vi "AB_Get Current VI Settings.vi"(11 "linkerInfo":T4) -> (3 "sourceProperties":T1[](array[typedef]))   [LabVIEW 2020]
uses:
  <vilib>/Utility/lvfile.llb/LVFileType.ctl
  <vilib>/AppBuilder/AB_Source_Properties.ctl
  <vilib>/AppBuilder/AB_Source_Property_Type.ctl
  <vilib>/AppBuilder/AB_Source_Property_WindowBehavior.ctl
  <vilib>/AppBuilder/AB_Source_Property_WindowRunTimePosition.ctl
  <vilib>/Utility/lvfile.llb/NI_FileType.lvlib
panel:
  in  "use hints for keep panel? (T)":bool=TRUE
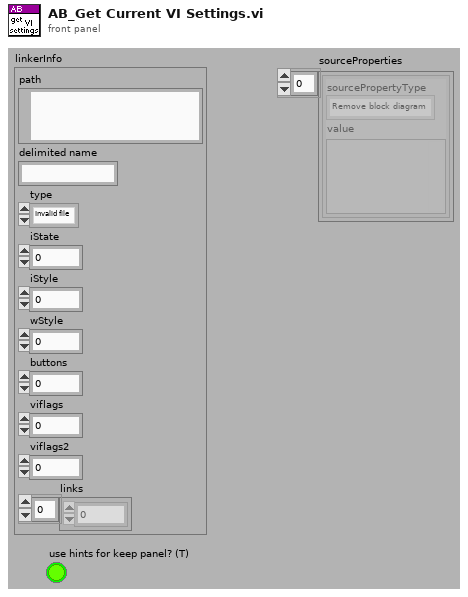
[diagram p1: front panel]
types:
  T1 = typedef "AB_Source_Properties.ctl" = cluster{"sourcePropertyType":T2, "value":variant}
  T2 = typedef "AB_Source_Property_Type.ctl" = enum16{"Remove block diagram", "Remove front panel", "Password", "Window has title bar", "Show menu bar", "Show vertical scroll bar", "Show horizontal scroll bar", "Show toolbar", "Show Abort button", "Show fp when called", "Window behavior", "Allow user to close window", "Window run-time position", "Run when opened", "Allow debugging", "Auto error handling", "Generate guard code", "Use stack variables", "Expression folding", "Integer only", "Inline subVI"}
  T3 = typedef "NI_FileType.lvlib/LVFileType.ctl" = enum32{"Invalid file", "Unknown type", "Instrument", "Control", "Polymorphic VI", "Project", "Library", "LVClass", "XControl", "XNode", "Shared library", ".NET assembly", "ActiveX interface", "CIN", "Run-time menu", "Palette menu", "Help file", "LLB", "XNode Edit Dependency", "Class Private Data Control", "Statechart", "MathScript .m file", "Ladder Diagram", "LVLibp", "XNode Build Dependency"}
  T4 = cluster{"path":path, "delimited name":string, "type":T3, "iState":u32, "iStyle":u16, "wStyle":u16, "buttons":u16, "viflags":u32, "viflags2":u32, "links":u32[]}
  T5 = typedef "AB_Source_Property_WindowBehavior.ctl" = enum16{"Default", "Floating", "Modal"}
  T6 = typedef "AB_Source_Property_WindowRunTimePosition.ctl" = enum16{"Unchanged", "Centered", "Maximized", "Minimized"}
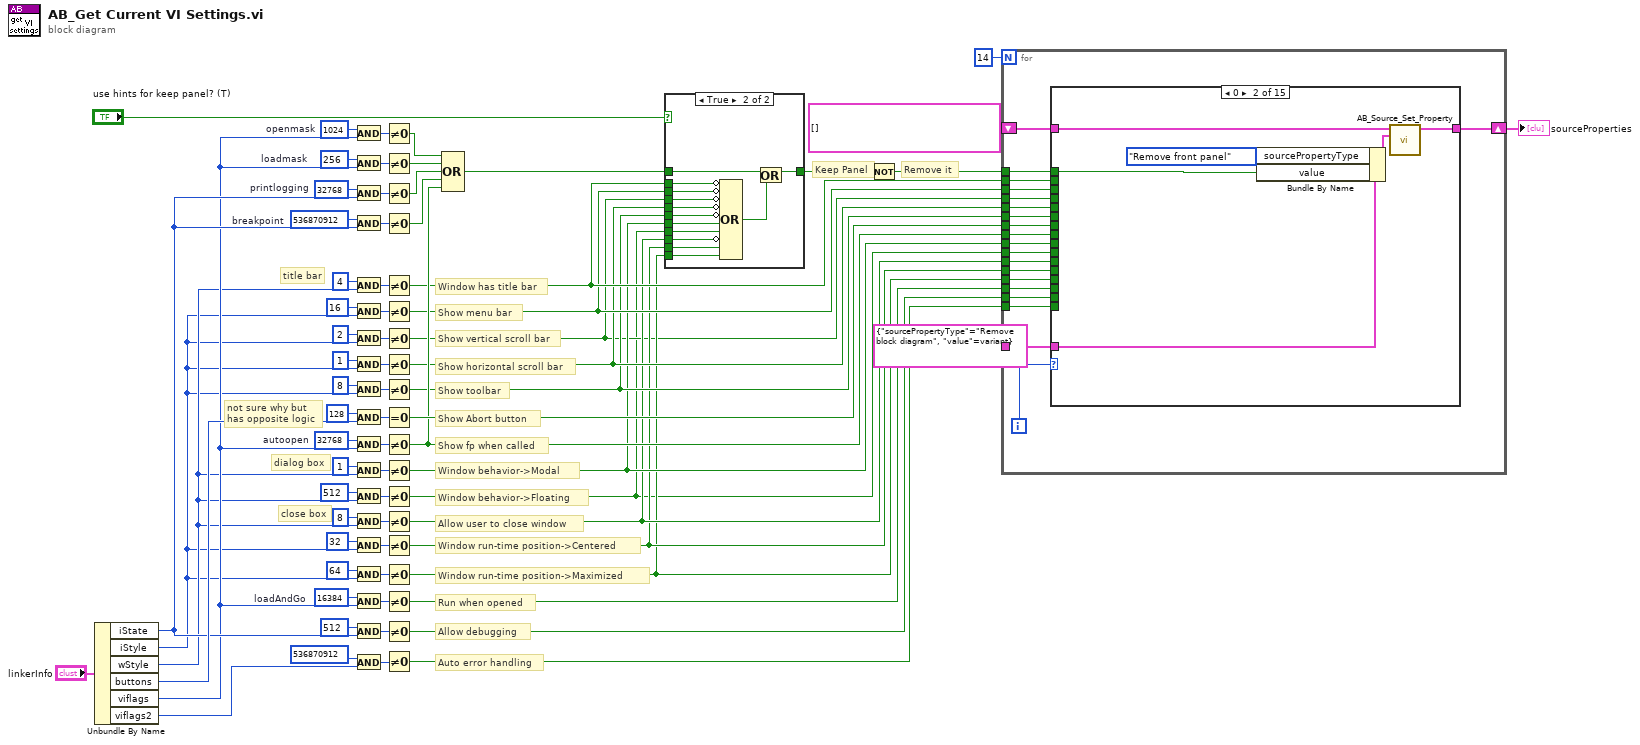
[diagram p0: block diagram]
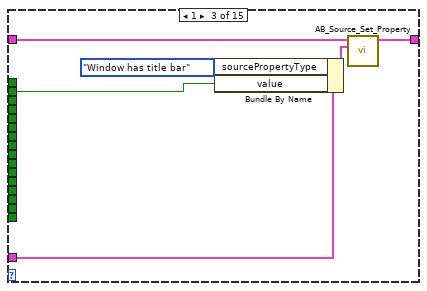
[diagram p3: hidden frame]
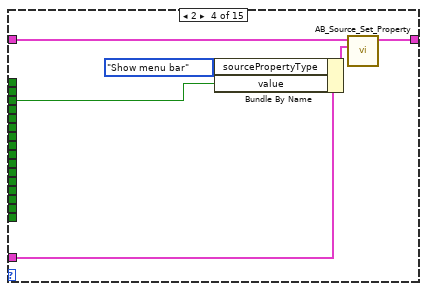
[diagram p4: hidden frame]
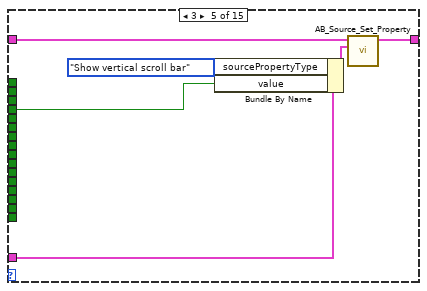
[diagram p5: hidden frame]
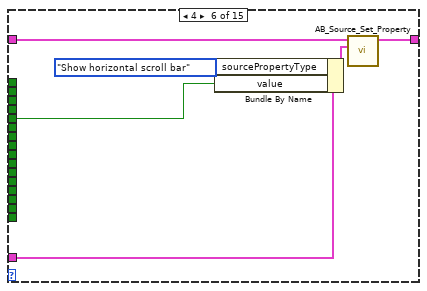
[diagram p6: hidden frame]
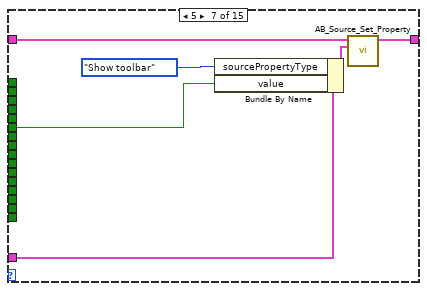
[diagram p7: hidden frame]
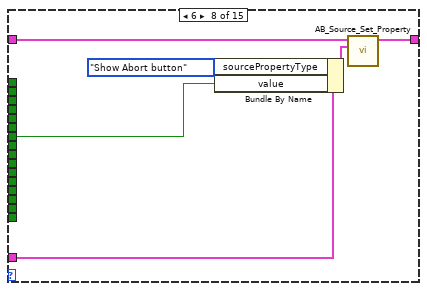
[diagram p8: hidden frame]
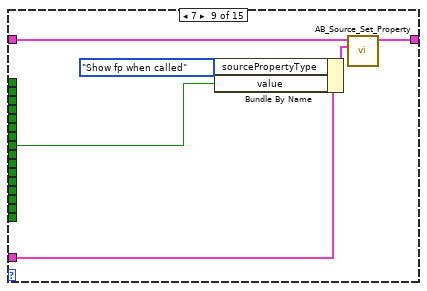
[diagram p9: hidden frame]
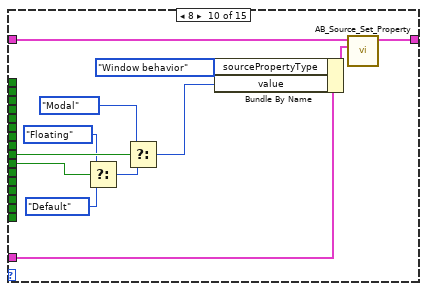
[diagram p10: hidden frame]
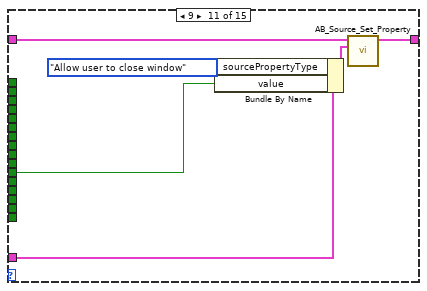
[diagram p11: hidden frame]
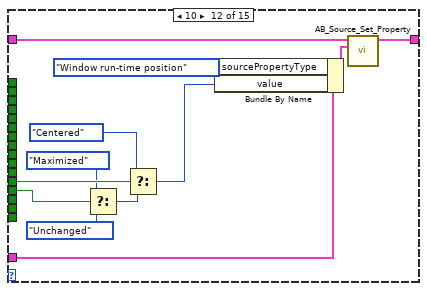
[diagram p12: hidden frame]
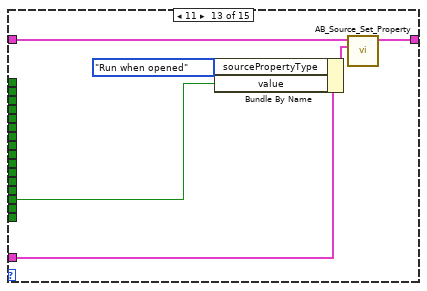
[diagram p13: hidden frame]
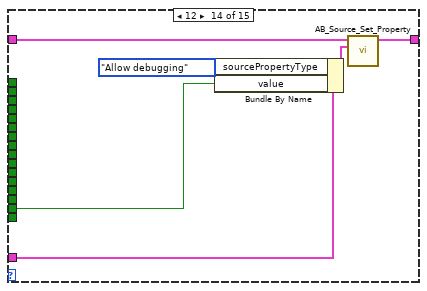
[diagram p14: hidden frame]
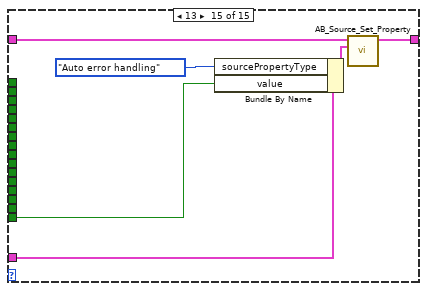
[diagram p15: hidden frame]
diagram:
  w35 = u32 16384  # loadAndGo
  w37 = u32 1024  # openmask
  w42 = u32 536870912  # breakpoint
  w44 = u32 32768  # printlogging
  w47 = u32 256  # loadmask
  w69 = u32 32768  # autoopen
  # "not sure why but has opposite logic"
  # "Auto error handling"
  # "Allow debugging"
  # "Run when opened"
  # "Window run-time position->Maximized"
  # "Window run-time position->Centered"
  # "Allow user to close window"
  # "Window behavior->Floating"
  # "Show fp when called"
  # "Show Abort button"
  # "Show toolbar"
  # "Show horizontal scroll bar"
  # "Show vertical scroll bar"
  # "Show menu bar"
  # "Window has title bar"
  # "Window behavior->Modal"
  # "Remove it"
  # "Keep Panel"
  # "title bar"
  # "close box"
  # "dialog box"
  n1 = Unbundle By Name("linkerInfo") -> ("iState"=w39:u32, "iStyle"=w13:u16, "wStyle"=w18:u16, "buttons"=w63:u16, "viflags"=w33:u32, "viflags2"=w30:u32)
  n2 = And(x=w37, y=w33) -> (x .and. y?=w38:u32)
  n3 = And(x=w47, y=w33) -> (x .and. y?=w48:u32)
  n4 = And(x=w44, y=w39) -> (x .and. y?=w45:u32)
  n5 = And(x=w42, y=w39) -> (x .and. y?=w41:u32)
  n6 = And(x=u16 4, y=w18) -> (x .and. y?=w60:u16)
  n7 = And(x=u16 16, y=w13) -> (x .and. y?=w57:u16)
  n8 = And(x=u16 2, y=w13) -> (x .and. y?=w23:u16)
  n9 = And(x=u16 1, y=w13) -> (x .and. y?=w53:u16)
  n10 = And(x=u16 8, y=w13) -> (x .and. y?=w56:u16)
  n11 = And(x=u16 128, y=w63) -> (x .and. y?=w67:u16)
  n12 = And(x=w69, y=w33) -> (x .and. y?=w68:u32)
  n13 = And(x=u16 1, y=w18) -> (x .and. y?=w66:u16)
  n14 = And(x=u16 512, y=w18) -> (x .and. y?=w19:u16)
  n15 = And(x=u16 8, y=w18) -> (x .and. y?=w61:u16)
  n16 = And(x=u16 32, y=w13) -> (x .and. y?=w52:u16)
  n17 = And(x=u16 64, y=w13) -> (x .and. y?=w49:u16)
  n18 = And(x=w35, y=w33) -> (x .and. y?=w34:u32)
  n19 = And(x=u32 512, y=w39) -> (x .and. y?=w70:u32)
  n20 = And(x=u32 536870912, y=w30) -> (x .and. y?=w29:u32)
  n21 = Not Equal To 0?(x=w38) -> (x != 0?=w36:bool)
  n22 = Not Equal To 0?(x=w48) -> (x != 0?=w46:bool)
  n23 = Not Equal To 0?(x=w45) -> (x != 0?=w43:bool)
  n24 = Not Equal To 0?(x=w41) -> (x != 0?=w40:bool)
  n25 = Not Equal To 0?(x=w60) -> (x != 0?=w10:bool)
  n26 = Not Equal To 0?(x=w57) -> (x != 0?=w9:bool)
  n27 = Not Equal To 0?(x=w23) -> (x != 0?=w2:bool)
  n28 = Not Equal To 0?(x=w53) -> (x != 0?=w8:bool)
  n29 = Not Equal To 0?(x=w56) -> (x != 0?=w7:bool)
  n30 = Equal To 0?(x=w67) -> (x = 0?=w21:bool)
  n31 = Not Equal To 0?(x=w68) -> (x != 0?=w14:bool)
  n32 = Not Equal To 0?(x=w66) -> (x != 0?=w6:bool)
  n33 = Not Equal To 0?(x=w19) -> (x != 0?=w1:bool)
  n34 = Not Equal To 0?(x=w61) -> (x != 0?=w5:bool)
  n35 = Not Equal To 0?(x=w52) -> (x != 0?=w4:bool)
  n36 = Not Equal To 0?(x=w49) -> (x != 0?=w3:bool)
  n37 = Not Equal To 0?(x=w34) -> (x != 0?=w15:bool)
  n38 = Not Equal To 0?(x=w70) -> (x != 0?=w17:bool)
  n39 = Not Equal To 0?(x=w29) -> (x != 0?=w16:bool)
  n40 = Compound Arithmetic op=OR(w36, w46, w43, w40, w14) -> (w26:bool)
  n41 = case shown="True" "use hints for keep panel? (T)" {
    tunnel: w26 -> [w73 w85]
    tunnel: [w73 w84] -> w25
    tunnel: w3 -> [_ w83]
    tunnel: w4 -> [_ w82]
    tunnel: w10 -> [_ w81]
    tunnel: w9 -> [_ w80]
    tunnel: w8 -> [_ w77]
    tunnel: w7 -> [_ w79]
    tunnel: w6 -> [_ w78]
    tunnel: w5 -> [_ w75]
    tunnel: w2 -> [_ w76]
    tunnel: w1 -> [_ w74]
    frame False {
    }
    frame True {
      n42 = Compound Arithmetic op=OR(invert w81, invert w80, invert w76, invert w77, invert w79, w78, w74, invert w75, w82, w83) -> (w86:bool)
      n43 = Or(x=w85, y=w86) -> (x .or. y?=w84:bool)
    }
  }
  n44 = Not(x=w25) -> (.not. x?=w24:bool)
  n45 = for {
    N: 14 -> [_]
    shift-right: [w105] -> w12
    shift-left: T1[] [] ("sourceProperties out") -> [w104]
    tunnel: T1 {"sourcePropertyType"=enum."Remove block diagram", "value"=variant} ("sourceProperty") -> [w103]
    tunnel: w24 -> [w102]
    tunnel: w10 -> [w101]
    tunnel: w9 -> [w100]
    tunnel: w2 -> [w99]
    tunnel: w8 -> [w98]
    tunnel: w7 -> [w97]
    tunnel: w21 -> [w96]
    tunnel: w14 -> [w95]
    tunnel: w4 -> [w94]
    tunnel: w3 -> [w93]
    tunnel: w5 -> [w92]
    tunnel: w6 -> [w91]
    tunnel: w1 -> [w90]
    tunnel: w15 -> [w89]
    tunnel: w17 -> [w88]
    tunnel: w16 -> [w87]
    i -> [w106]
    n46 = case shown="0" w106 {
      tunnel: [w107 w113 w119 w125 w131 w137 w143 w149 w155 w167 w173 w185 w191 w197 w203] -> w105
      tunnel: w104 -> [w107 w112 w118 w124 w130 w136 w142 w148 w154 w166 w172 w184 w190 w196 w202]
      tunnel: w103 -> [_ w111 w117 w123 w129 w135 w141 w147 w153 w165 w171 w183 w189 w195 w201]
      tunnel: w102 -> [_ w108 _ _ _ _ _ _ _ _ _ _ _ _ _]
      tunnel: w101 -> [_ _ w114 _ _ _ _ _ _ _ _ _ _ _ _]
      tunnel: w100 -> [_ _ _ w120 _ _ _ _ _ _ _ _ _ _ _]
      tunnel: w99 -> [_ _ _ _ w126 _ _ _ _ _ _ _ _ _ _]
      tunnel: w98 -> [_ _ _ _ _ w132 _ _ _ _ _ _ _ _ _]
      tunnel: w97 -> [_ _ _ _ _ _ w138 _ _ _ _ _ _ _ _]
      tunnel: w96 -> [_ _ _ _ _ _ _ w144 _ _ _ _ _ _ _]
      tunnel: w95 -> [_ _ _ _ _ _ _ _ w150 _ _ _ _ _ _]
      tunnel: w94 -> [_ _ _ _ _ _ _ _ _ _ _ w180 _ _ _]
      tunnel: w93 -> [_ _ _ _ _ _ _ _ _ _ _ w179 _ _ _]
      tunnel: w92 -> [_ _ _ _ _ _ _ _ _ _ w168 _ _ _ _]
      tunnel: w91 -> [_ _ _ _ _ _ _ _ _ w160 _ _ _ _ _]
      tunnel: w90 -> [_ _ _ _ _ _ _ _ _ w156 _ _ _ _ _]
      tunnel: w89 -> [_ _ _ _ _ _ _ _ _ _ _ _ w186 _ _]
      tunnel: w88 -> [_ _ _ _ _ _ _ _ _ _ _ _ _ w192 _]
      tunnel: w87 -> [_ _ _ _ _ _ _ _ _ _ _ _ _ _ w198]
      frame Default {
      }
      frame 0 {
        n47 = Bundle By Name(cluster=w111, "sourcePropertyType"=AB_Source_Property_Type."Remove front panel", "value"=w108) -> (w110:T1)
        n48 = call <vilib>:"AB_Source_Set_Property.vi"("sourceProperty"=w110, "sourceProperties in"=w112) -> ("sourceProperties out"=w113:T1[])  [unwired: 7 in, 2 out]
      }
      frame 1 {
        n49 = Bundle By Name(cluster=w117, "sourcePropertyType"=AB_Source_Property_Type."Window has title bar", "value"=w114) -> (w116:T1)
        n50 = call <vilib>:"AB_Source_Set_Property.vi"("sourceProperty"=w116, "sourceProperties in"=w118) -> ("sourceProperties out"=w119:T1[])  [unwired: 7 in, 2 out]
      }
      frame 2 {
        n51 = Bundle By Name(cluster=w123, "sourcePropertyType"=AB_Source_Property_Type."Show menu bar", "value"=w120) -> (w122:T1)
        n52 = call <vilib>:"AB_Source_Set_Property.vi"("sourceProperty"=w122, "sourceProperties in"=w124) -> ("sourceProperties out"=w125:T1[])  [unwired: 7 in, 2 out]
      }
      frame 3 {
        n53 = Bundle By Name(cluster=w129, "sourcePropertyType"=AB_Source_Property_Type."Show vertical scroll bar", "value"=w126) -> (w128:T1)
        n54 = call <vilib>:"AB_Source_Set_Property.vi"("sourceProperty"=w128, "sourceProperties in"=w130) -> ("sourceProperties out"=w131:T1[])  [unwired: 7 in, 2 out]
      }
      frame 4 {
        n55 = Bundle By Name(cluster=w135, "sourcePropertyType"=AB_Source_Property_Type."Show horizontal scroll bar", "value"=w132) -> (w134:T1)
        n56 = call <vilib>:"AB_Source_Set_Property.vi"("sourceProperty"=w134, "sourceProperties in"=w136) -> ("sourceProperties out"=w137:T1[])  [unwired: 7 in, 2 out]
      }
      frame 5 {
        n57 = Bundle By Name(cluster=w141, "sourcePropertyType"=AB_Source_Property_Type."Show toolbar", "value"=w138) -> (w140:T1)
        n58 = call <vilib>:"AB_Source_Set_Property.vi"("sourceProperty"=w140, "sourceProperties in"=w142) -> ("sourceProperties out"=w143:T1[])  [unwired: 7 in, 2 out]
      }
      frame 6 {
        n59 = Bundle By Name(cluster=w147, "sourcePropertyType"=AB_Source_Property_Type."Show Abort button", "value"=w144) -> (w146:T1)
        n60 = call <vilib>:"AB_Source_Set_Property.vi"("sourceProperty"=w146, "sourceProperties in"=w148) -> ("sourceProperties out"=w149:T1[])  [unwired: 7 in, 2 out]
      }
      frame 7 {
        n61 = Bundle By Name(cluster=w153, "sourcePropertyType"=AB_Source_Property_Type."Show fp when called", "value"=w150) -> (w152:T1)
        n62 = call <vilib>:"AB_Source_Set_Property.vi"("sourceProperty"=w152, "sourceProperties in"=w154) -> ("sourceProperties out"=w155:T1[])  [unwired: 7 in, 2 out]
      }
      frame 8 {
        n63 = Select(t=AB_Source_Property_WindowBehavior."Floating" ("windowBehavior"), s=w156, f=AB_Source_Property_WindowBehavior."Default" ("windowBehavior")) -> (s? t:f=w162:T5)
        n64 = Select(t=AB_Source_Property_WindowBehavior."Modal" ("windowBehavior"), s=w160, f=w162) -> (s? t:f=w161:T5)
        n65 = Bundle By Name(cluster=w165, "sourcePropertyType"=AB_Source_Property_Type."Window behavior", "value"=w161) -> (w164:T1)
        n66 = call <vilib>:"AB_Source_Set_Property.vi"("sourceProperty"=w164, "sourceProperties in"=w166) -> ("sourceProperties out"=w167:T1[])  [unwired: 7 in, 2 out]
      }
      frame 9 {
        n67 = Bundle By Name(cluster=w171, "sourcePropertyType"=AB_Source_Property_Type."Allow user to close window", "value"=w168) -> (w170:T1)
        n68 = call <vilib>:"AB_Source_Set_Property.vi"("sourceProperty"=w170, "sourceProperties in"=w172) -> ("sourceProperties out"=w173:T1[])  [unwired: 7 in, 2 out]
      }
      frame 10 {
        n69 = Select(t=AB_Source_Property_WindowRunTimePosition."Maximized" ("windowRunTimePosition"), s=w179, f=AB_Source_Property_WindowRunTimePosition."Unchanged" ("windowRunTimePosition")) -> (s? t:f=w178:T6)
        n70 = Select(t=AB_Source_Property_WindowRunTimePosition."Centered" ("windowRunTimePosition"), s=w180, f=w178) -> (s? t:f=w175:T6)
        n71 = Bundle By Name(cluster=w183, "sourcePropertyType"=AB_Source_Property_Type."Window run-time position", "value"=w175) -> (w182:T1)
        n72 = call <vilib>:"AB_Source_Set_Property.vi"("sourceProperty"=w182, "sourceProperties in"=w184) -> ("sourceProperties out"=w185:T1[])  [unwired: 7 in, 2 out]
      }
      frame 11 {
        n73 = Bundle By Name(cluster=w189, "sourcePropertyType"=AB_Source_Property_Type."Run when opened", "value"=w186) -> (w188:T1)
        n74 = call <vilib>:"AB_Source_Set_Property.vi"("sourceProperty"=w188, "sourceProperties in"=w190) -> ("sourceProperties out"=w191:T1[])  [unwired: 7 in, 2 out]
      }
      frame 12 {
        n75 = Bundle By Name(cluster=w195, "sourcePropertyType"=AB_Source_Property_Type."Allow debugging", "value"=w192) -> (w194:T1)
        n76 = call <vilib>:"AB_Source_Set_Property.vi"("sourceProperty"=w194, "sourceProperties in"=w196) -> ("sourceProperties out"=w197:T1[])  [unwired: 7 in, 2 out]
      }
      frame 13 {
        n77 = Bundle By Name(cluster=w201, "sourcePropertyType"=AB_Source_Property_Type."Auto error handling", "value"=w198) -> (w200:T1)
        n78 = call <vilib>:"AB_Source_Set_Property.vi"("sourceProperty"=w200, "sourceProperties in"=w202) -> ("sourceProperties out"=w203:T1[])  [unwired: 7 in, 2 out]
      }
    }
  }
  "sourceProperties" <- w12
